vi "Fpga_v8.vi"() -> ()   [LabVIEW 2015]
uses:
  <vilib>/rvi/Emulation/niFpgaGetClockAttributes.vi
  <vilib>/rvi/Emulation/niFpgaSctlEmulationGetInTimedLoop.vi
  <vilib>/rvi/Emulation/niFpgaEmulationReportErrorSimple.vi
  <vilib>/rvi/eio/common/nirviEmuTemplateMethod_errors.vi
  <vilib>/rvi/Emulation/niFpgaCriticalErrorInLSC.vi
  <vilib>/eio/EIONode/EIONode.xnode
panel:
  out "x+y":i32
  in  "stop inner loop":bool
  out "fixed-point":fxp<+/-,32,32>
  out "no use":u32
  out "snap chat":u32
  in  "Gradual increase loop speed (uSec)":u32 caption="Count(uSec)"
  out "x-y":u32
  in  "start":bool
  in  "stop":bool
  out "Mod2/DIO6_B":bool
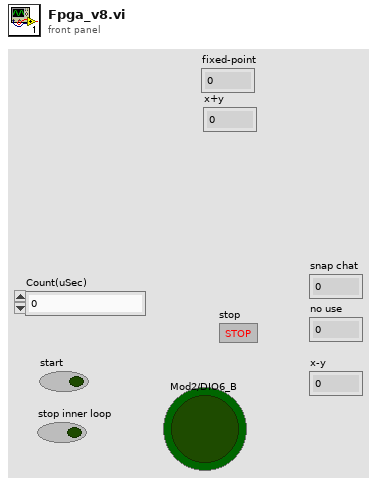
[diagram p1: front panel]
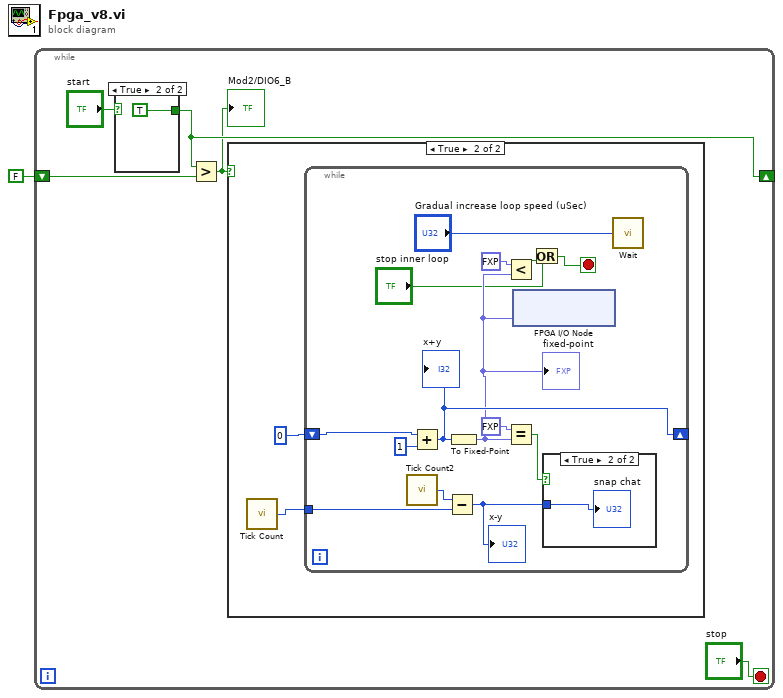
[diagram p0: block diagram]
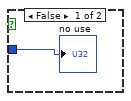
[diagram p3: hidden frame]
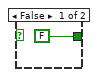
[diagram p4: hidden frame]
diagram:
  n1 = while {
    shift-right: [w5] -> _
    shift-left: FALSE -> [w6]
    stop <- "stop" stop-if-true
    n2 = case shown="True" "start" {
      tunnel: [FALSE ("Mod2/DIO6") TRUE ("Mod2/DIO6")] -> w5
      frame False {
      }
      frame True {
      }
    }
    n3 = Greater?(x=w5, y=w6) -> (0:w2:bool)
    "Mod2/DIO6_B" <- w2
    n4 = case shown="True" w2 {
      frame False {
      }
      frame True {
        n5 = call "Tick Count"() -> ("Tick Count(mSec)"=w8:u32)
        n6 = while {
          tunnel: w8 -> [w21]
          shift-right: [w13] -> _
          shift-left: 0 ("x") -> [w14]
          stop <- w10 stop-if-true
          n7 = call "Tick Count2"() -> ("Tick Count(mSec)"=w22:u32)
          n8 = Add(x=w14, y=1 ("x")) -> (x+y=w13:i32)
          "x+y" <- w13
          n9 = Subtract(x=w22, y=w21) -> (x-y=w18:u32)
          "x-y" <- w18
          n10 = To Fixed-Point(number=w13) -> (fixed-point=w12:fxp<+/-,32,32>)  [unwired: 1 in]
          "fixed-point" <- w12
          n11 = Less?(x=fxp<+,32,32> 8.0, y=w12) -> (x < y?=w11:bool)
          n12 = Equal?(x=fxp<+,64,32> 6.0, y=w12) -> (x = y?=w19:bool)
          n13 = xnode "FPGA I/O Node"("Mod4/AO0"=w12) -> ()  [unwired: 1 in, 1 out]
          n14 = Or(x="stop inner loop", y=w11) -> (x .or. y?=w10:bool)
          n15 = case shown="True" w19 {
            tunnel: w18 -> [w23 w24]
            frame False {
              "no use" <- w23
            }
            frame True {
              "snap chat" <- w24
            }
          }
          n16 = call "Wait"("Count(uSec)"="Gradual increase loop speed (uSec)") -> ()  [unwired: 1 out]
        }
      }
    }
  }
